vi "write multiple registers.vi"(8 "error in (no error)":errorcluster, 9 "register values":u16[](array[numeric]) format="%.0x", 10 "addresses":u16[](array[numeric]) format="%.0x", 11 "CL57RS in":refnum<class "CL57RS.lvclass">) -> (0 "error out":errorcluster, 3 "CL57RS out":refnum<class "CL57RS.lvclass">)   [LabVIEW 2025, in "Motor.lvlib" / "CL57RS.lvclass"]
uses:
  CL57RS.lvclass
  CL57RS.lvclass/CL57RS.ctl
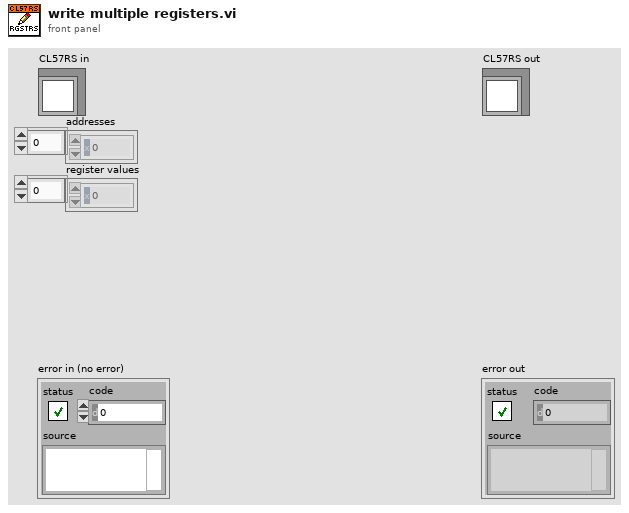
[diagram p1: front panel]
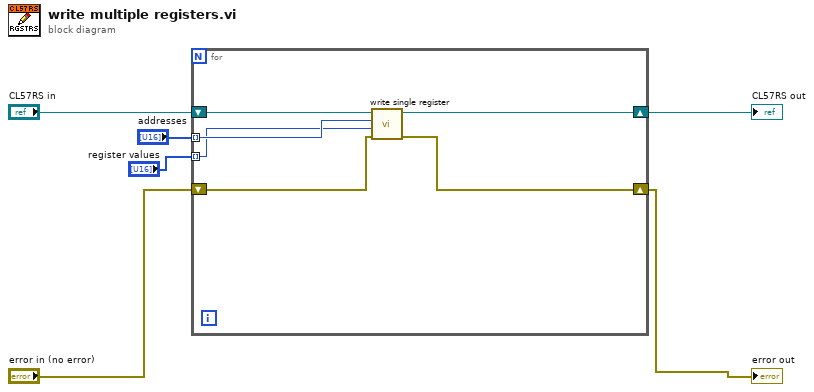
[diagram p0: block diagram]
diagram:
  n1 = for {
    shift-right: [w11] -> w3
    shift-left: "CL57RS in" -> [w10]
    shift-right: [w12] -> w1
    shift-left: "error in (no error)" -> [w7]
    tunnel: "addresses" -> [w9] mode=indexing
    tunnel: "register values" -> [w8] mode=indexing
    n2 = call "write single register.vi"("error in (no error)"=w7, "register to write"=w8, "address"=w9, "CL57RS in"=w10) -> ("error out"=w12:errorcluster, "CL57RS out"=w11:refnum<class "CL57RS.lvclass">)  [unwired: 6 in]
  }
  "error out" <- w1
  "CL57RS out" <- w3
